vi "Agilent PWM Config Test.vi"(8 "error in (no error)":errorcluster, 10 "Configuration":T2={"BusType"=enum."GPIB", "GPIB Bus"=0, "GPIB Address"=16, "IP"=0, "COM"=1, "Baud Rate"=enum."9600", "USB Device"=0, "Instrument S\\N"="", "SCIL Address"=16} {"USB Device" max=31 step=1}, 11 "Str Refnum":refnum<vi>) -> (0 "error out":errorcluster, 3 "Agilent PWM":T1)   [LabVIEW 2011]
uses:
  PWM Configuration.ctl
  TypeDefs/Agilent PWM Instrument Info.ctl
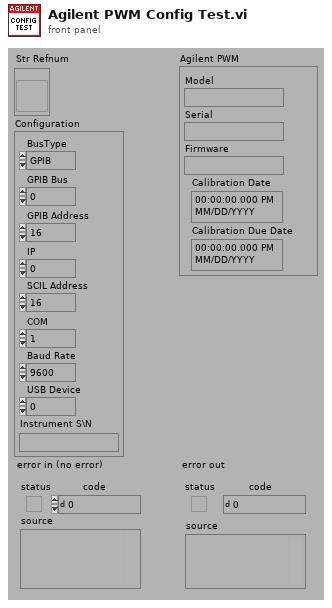
[diagram p1: front panel]
types:
  T1 = typedef "Agilent PWM Instrument Info.ctl" = cluster{"Model":string, "Serial":string, "Firmware":string, "Calibration Date":timestamp, "Calibration Due Date":timestamp}
  T2 = typedef "PWM Configuration.ctl" = cluster{"BusType":enum32{"GPIB", "LAN/IP", "Serial", "USB"}, "GPIB Bus":i32, "GPIB Address":i32, "IP":u32, "COM":i32, "Baud Rate":enum32{"300", "600", "1200", "2400", "4800", "9600"}, "USB Device":u32, "Instrument S\\N":string, "SCIL Address":i32}
  T3 = enum32{"300", "600", "1200", "2400", "4800", "9600"}
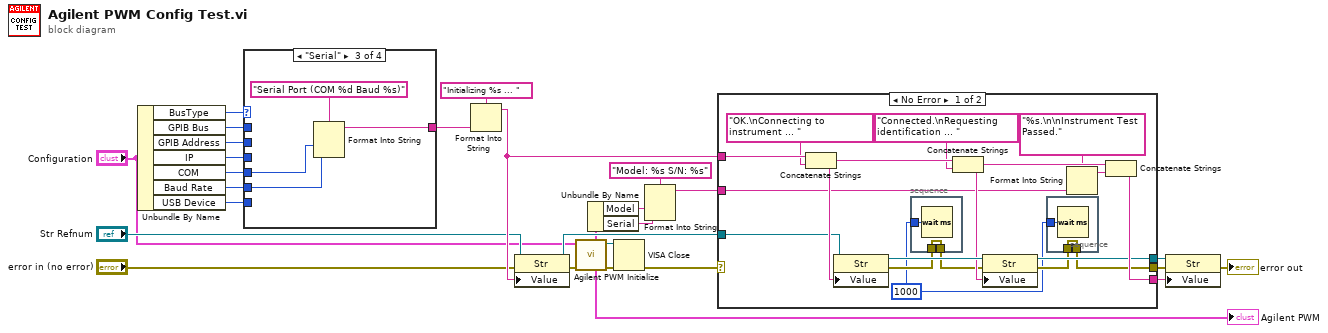
[diagram p0: block diagram]
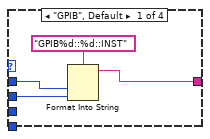
[diagram p2: hidden frame]
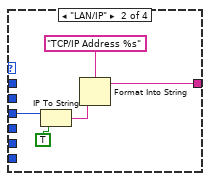
[diagram p3: hidden frame]
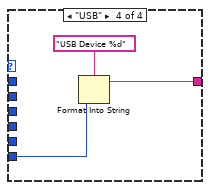
[diagram p4: hidden frame]
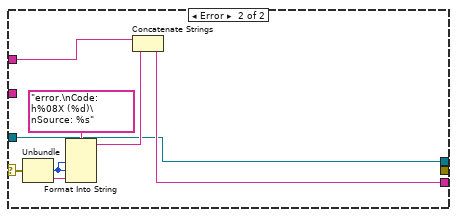
[diagram p5: hidden frame]
diagram:
  n1 = Unbundle By Name("Configuration") -> ("BusType"=w10:enum32{"GPIB", "LAN/IP", "Serial", "USB"}, "GPIB Bus"=w9:i32, "GPIB Address"=w8:i32, "IP"=w7:u32, "COM"=w6:i32, "Baud Rate"=w5:T3, "USB Device"=w4:u32)
  n2 = case shown="\"Serial\"" w10 {
    tunnel: w9 -> [w30 _ _ _]
    tunnel: w8 -> [w29 _ _ _]
    tunnel: w7 -> [_ w35 _ _]
    tunnel: w6 -> [_ _ w39 _]
    tunnel: [w28 w32 w38 w42] -> w2
    tunnel: w5 -> [_ _ w37 _]
    tunnel: w4 -> [_ _ _ w41]
    frame "GPIB", Default {
      n3 = Format Into String(format string="GPIB%d::%d::INST", w30, w29) -> (resulting string=w28:string)  [unwired: 2 in, 1 out]
    }
    frame "LAN/IP" {
      n4 = IP To String(1:TRUE, 2:w35) -> (0:w34:string)
      n5 = Format Into String(format string="TCP/IP Address %s", w34) -> (resulting string=w32:string)  [unwired: 2 in, 1 out]
    }
    frame "Serial" {
      n6 = Format Into String(format string="Serial Port (COM %d Baud %s)", w39, w37) -> (resulting string=w38:string)  [unwired: 2 in, 1 out]
    }
    frame "USB" {
      n7 = Format Into String(format string="USB Device %d", w41) -> (resulting string=w42:string)  [unwired: 2 in, 1 out]
    }
  }
  n8 = Format Into String(format string="Initializing %s ... ", w2) -> (resulting string=w26:string)  [unwired: 2 in, 1 out]
  n9 = property class="Str"(reference="Str Refnum", error in="error in (no error)", "Value"=w26) -> (reference out=w12:refnum<vi>, error out=w24:errorcluster)
  n10 = call "Agilent PWM Initialize.vi"("error in (no error)"=w24, "Configuration"="Configuration") -> ("error out"=w21:errorcluster, "VISA Resource Name"=w19:refnum<visa-resource-name>, "Agilent PWM"=w1:T1)  [unwired: 7 out]
  "Agilent PWM" <- w1
  n11 = Unbundle By Name(w1) -> ("Model"=w22:string, "Serial"=w11:string)
  n12 = VISA Close(VISA resource name=w19, error in (no error)=w21) -> (error out=w20:errorcluster)
  n13 = Format Into String(format string="Model: %s S/N: %s" ("Return Model and Serial #"), w22, w11) -> (resulting string=w18:string)  [unwired: 2 in, 1 out]
  n14 = case shown="No Error" w20 {
    selector: w20 -> [_ w70]
    tunnel: w26 -> [w59 w72]
    tunnel: w12 -> [w54 w65]
    tunnel: w18 -> [w51 _]
    tunnel: [w50 w66] -> w17
    tunnel: [w49 w65] -> w15
    tunnel: [w45 _] -> w14
    frame No Error {
      w44 = u32 1000 ("milliseconds to wait")
      n15 = Concatenate Strings(w59, "OK.\nConnecting to instrument ... ") -> (w57:string)
      n16 = property class="Str"(reference=w54, "Value"=w57) -> (reference out=w60:refnum<vi>, error out=w48:errorcluster)  [unwired: 1 in]
      n17 = stacked-sequence {
        tunnel: w44 -> [w64]
        tunnel: w48 -> [w63]
        tunnel: [w63] -> w47
        frame #0 {
          n18 = Wait (ms)(milliseconds to wait=w64) -> ()  [unwired: 1 out]
        }
      }
      n19 = Concatenate Strings(w57, "Connected.\nRequesting identification ... ") -> (w55:string)
      n20 = property class="Str"(reference=w60, error in=w47, "Value"=w55) -> (reference out=w49:refnum<vi>, error out=w46:errorcluster)
      n21 = stacked-sequence {
        tunnel: w44 -> [w62]
        tunnel: w46 -> [w61]
        tunnel: [w61] -> w45
        frame #0 {
          n22 = Wait (ms)(milliseconds to wait=w62) -> ()  [unwired: 1 out]
        }
      }
      n23 = Format Into String(format string="%s.\n\nInstrument Test Passed.", w51) -> (resulting string=w52:string)  [unwired: 2 in, 1 out]
      n24 = Concatenate Strings(w55, w52) -> (w50:string)
    }
    frame Error {
      n25 = Unbundle(w70) -> ("code"=w69:i32, "source"=w68:string)  [unwired: 1 out]
      n26 = Format Into String(format string="error.\nCode:  h%08X (%d)\nSource: %s", w69, w69, w68) -> (resulting string=w67:string)  [unwired: 2 in, 1 out]
      n27 = Concatenate Strings(w72, w67) -> (w66:string)
    }
  }
  n28 = property class="Str"(reference=w15, error in=w14, "Value"=w17) -> (error out=→"error out":errorcluster)  [unwired: 1 out]
